vi "A Star Plan.vi"(8 "error in (no error)":errorcluster, 9 "goal reference":refnum<data-value>, 10 "start reference":refnum<data-value>, 11 "map reference in":refnum<data-value>) -> (0 "error out":errorcluster, 1 "no valid path exists":bool, 2 "path references":refnum<data-value>[](array[refnum]), 4 "path cost":dbl)   [LabVIEW 2017, in "NI_Robotics_Navigation .lvlib"]
doc: "Plans a least-cost path through a static map to a <B>goal reference</B> within a map. Use this VI to return a single, optimal path."
uses:
  <vilib>/robotics/Navigation/NI_Robotics_Navigation .lvlib
  <vilib>/robotics/Navigation/shared/MapNode/AbstractAstarNode/NI_Robotics_AbstractAstarNode.lvclass
  c:/Program Files (x86)/National Instruments/LabVIEW 2017/vi.lib/robotics/Navigation/shared/MapNode/AbstractMapNode/NI_Robotics_AbstractMapNode.lvclass
  <vilib>/robotics/Navigation/shared/WorldMap/AbstractWorldMap/NI_Robotics_AbstractWorldMap.lvclass
  <vilib>/robotics/Navigation/shared/Priority Queue/Open List Element.ctl
  <vilib>/robotics/Navigation/shared/MapNode/AbstractMapNode/NI_Robotics_AbstractMapNode.lvclass
  <vilib>/robotics/Navigation/Astar/Visited List Element.ctl
  <vilib>/robotics/Navigation/shared/Priority Queue/NI_Robotics_Priority Queue.lvclass
panel:
  out "num states":i32
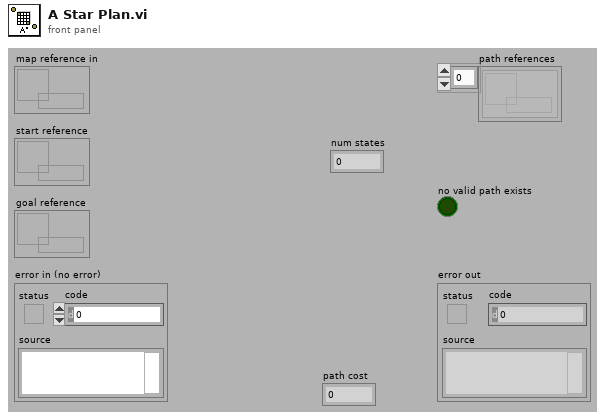
[diagram p1: front panel]
types:
  T1 = typedef "NI_Robotics_Priority Queue.lvclass/Open List Element.ctl" = cluster{"f":dbl, "g":dbl, "node Ref":refnum<data-value>}
  T2 = typedef "NI_Robotics_Navigation .lvlib/Visited List Element.ctl" = cluster{"Best cost to state":dbl, "Back pointer":refnum<data-value>}
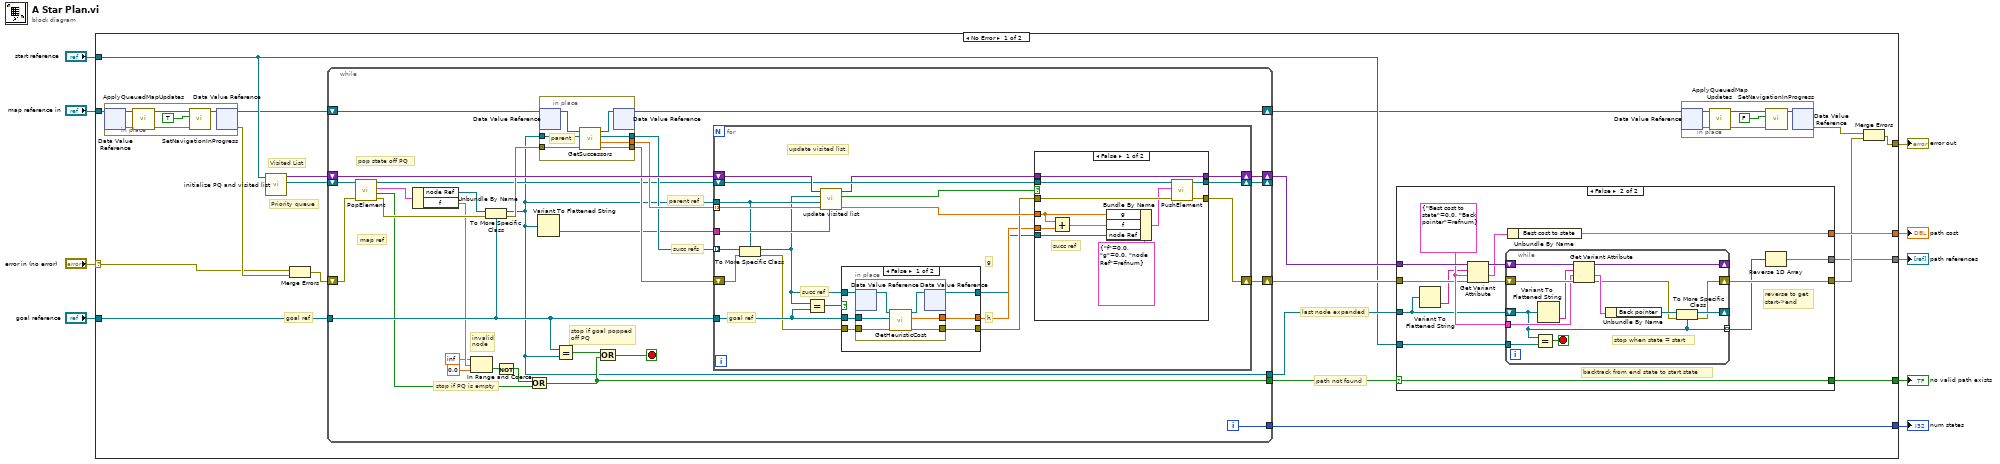
[diagram p0: block diagram]
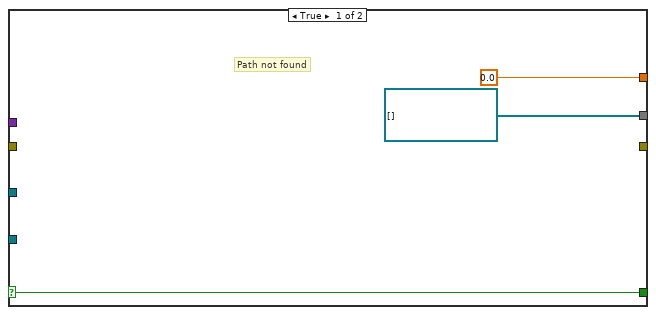
[diagram p2: hidden frame]
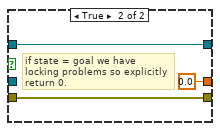
[diagram p3: hidden frame]
diagram:
  n1 = case shown="No Error" "error in (no error)" {
    selector: "error in (no error)" -> [w10 w158]
    tunnel: [w28 _] -> w9
    tunnel: "goal reference" -> [w23 _]
    tunnel: "start reference" -> [w22 _]
    tunnel: "map reference in" -> [w21 _]
    tunnel: [w15 w158] -> w5
    tunnel: [w13 _] -> w4
    tunnel: [w12 _] -> w3
    tunnel: [w11 _] -> w2
    frame No Error {
      # "goal ref"
      # "last node expanded"
      # "path not found"
      # "Priority queue"
      # "Visited List"
      n2 = in-place {
        n3 = in-place-dvr #1(w21) -> (w42:refnum<class "NI_Robotics_AbstractWorldMap.lvclass">, w41:errorcluster)
        n4 = call-dynamic "ApplyQueuedMapUpdates.vi"("error in (no error)"=w41, "AbstractWorldMap in"=w42) -> ("error out"=w38:errorcluster, "AbstractWorldMap out"=w40:refnum<class "NI_Robotics_AbstractWorldMap.lvclass">)  [unwired: 8 in]
        n5 = call-dynamic "SetNavigationInProgress.vi"("error in (no error)"=w38, "navigation in progress"=TRUE ("Navigation in Progress"), "AbstractWorldMap in"=w40) -> ("AbstractWorldMap out"=w39:refnum<class "NI_Robotics_AbstractWorldMap.lvclass">)  [unwired: 7 in, 1 out]
        n6 = in-place-dvr #1(w39) -> (w20:refnum<data-value>, w17:errorcluster)
      }
      n7 = call <vilib>:"initialize PQ and visited list.vi"("start state"=w22) -> ("Astar Open List out"=w24:refnum<class "NI_Robotics_Priority Queue.lvclass">, "visited list"=w30:variant)  [unwired: 9 out]
      n8 = Merge Errors(w10, w17) -> (w18:errorcluster)
      n9 = while {
        shift-right: [w97] -> _
        shift-left: w24 -> [w95]
        shift-right: [w99] -> w27
        shift-left: w30 -> [w101]
        tunnel: [w74] -> w26
        tunnel: w23 -> [w83]
        shift-right: [w98] -> w29
        shift-left: w18 -> [w94]
        tunnel: [w80] -> w25
        shift-right: [w82] -> w19
        shift-left: w20 -> [w84]
        tunnel: [w73] -> w12
        i -> [w73]
        stop <- w96 stop-if-true
        # "parent ref"
        # "invalid\nnode"
        # "map ref"
        # "succ refs"
        # "stop if goal popped\noff PQ"
        # "stop if PQ is empty"
        # "pop state off PQ"
        n10 = call <vilib>:"PopElement.vi"("error in (no error)"=w94, "Astar Open List in"=w95) -> ("error out"=w92:errorcluster, "empty"=w81:bool, "open list element"=w93:T1, "Astar Open List out"=w87:refnum<class "NI_Robotics_Priority Queue.lvclass">)  [unwired: 6 in]
        n11 = Unbundle By Name(w93) -> ("node Ref"=w85:refnum<data-value>, "f"=w79:dbl)
        n12 = In Range and Coerce(upper limit=inf, x=w79, lower limit=0.0) -> (In Range?=w75:bool)  [unwired: 1 out]
        n13 = To More Specific Class(target class=w83, reference=w85, error in=w92) -> (specific class reference=w74:refnum<data-value>, error out=w91:errorcluster)
        n14 = Not(x=w75) -> (.not. x?=w76:bool)
        n15 = Or(x=w76, y=w81) -> (x .or. y?=w80:bool)
        n16 = Variant To Flattened String(Variant=w74) -> (data string=w86:string)  [unwired: 1 out]
        n17 = in-place {
          in-place-border: w91 -> [w108]
          in-place-border: [w107] -> w90
          in-place-border: [w106] -> w89
          in-place-border: [w105] -> w88
          in-place-border: w74 -> [w102]
          # "parent"
          n18 = in-place-dvr #2(w84) -> (w104:refnum<class "NI_Robotics_AbstractWorldMap.lvclass">)  [unwired: 1 out]
          n19 = call-dynamic "GetSuccessors.vi"("error in (no error)"=w108, "AbstractMapNode Ref"=w102, "WorldMap in"=w104) -> ("error out"=w107:errorcluster, "EdgeCost"=w106:dbl[], "Successors"=w105:refnum<data-value>[], "WorldMap out"=w103:refnum<class "NI_Robotics_AbstractWorldMap.lvclass">)  [unwired: 5 in]
          n20 = in-place-dvr #2(w103) -> (w82:refnum<data-value>)  [unwired: 1 out]
        }
        n21 = Equal?(x=w83, y=w74) -> (x = y?=w100:bool)
        n22 = Or(x=w100, y=w80) -> (x .or. y?=w96:bool)
        n23 = for {
          shift-right: [w124] -> w97
          shift-left: w87 -> [w125]
          shift-right: [w109] -> w99
          shift-left: w101 -> [w128]
          tunnel: w88 -> [w122] mode=indexing
          tunnel: w89 -> [w118] mode=indexing
          tunnel: w86 -> [w119]
          tunnel: w83 -> [w113]
          shift-right: [w123] -> w98
          shift-left: w90 -> [w112]
          tunnel: w74 -> [w117]
          # "succ ref"
          # "goal ref"
          # "h"
          # "g"
          # "update visited list"
          n24 = To More Specific Class(target class=w117, reference=w122, error in=w112) -> (specific class reference=w114:refnum<data-value>, error out=w111:errorcluster)
          n25 = Equal?(x=w114, y=w113) -> (x = y?=w115:bool)
          n26 = call <vilib>:"update visited list.vi"("previous node string"=w119, "edge cost"=w118, "previous node"=w117, "current node"=w114, "visited list in"=w128) -> ("path cost"=w126:dbl, "discarded"=w127:bool, "visited list out"=w110:variant)  [unwired: 4 out]
          n27 = case shown="False" w115 {
            tunnel: w113 -> [w134 _]
            tunnel: w111 -> [w133 w142]
            tunnel: [w132 w142] -> w121
            tunnel: [w131 0.0 ("Hueristic Cost")] -> w120
            tunnel: w114 -> [w130 w143]
            tunnel: [w129 w143] -> w116
            frame False {
              n28 = in-place {
                in-place-border: w134 -> [w140]
                in-place-border: w133 -> [w139]
                in-place-border: [w138] -> w132
                in-place-border: [w137] -> w131
                n29 = in-place-dvr #3(w130) -> (w136:refnum<class "NI_Robotics_AbstractAstarNode.lvclass">)  [unwired: 1 out]
                n30 = call-dynamic "GetHeuristicCost.vi"("error in (no error)"=w139, "Goal NodeReference"=w140, "AbstractAstarNode in"=w136) -> ("error out"=w138:errorcluster, "hueristic cost"=w137:dbl, "AbstractAstarNode out"=w135:refnum<class "NI_Robotics_AbstractAstarNode.lvclass">)  [unwired: 6 in]
                n31 = in-place-dvr #3(w135) -> (w129:refnum<data-value>)  [unwired: 1 out]
              }
            }
            frame True {
              # "if state = goal we have locking problems so explicitly return 0."
            }
          }
          n32 = case shown="False" w127 {
            tunnel: w126 -> [w147 _]
            tunnel: w125 -> [w152 w156]
            tunnel: [w149 w156] -> w124
            tunnel: w120 -> [w148 _]
            tunnel: w116 -> [w153 _]
            tunnel: w121 -> [w151 w157]
            tunnel: [w150 w157] -> w123
            tunnel: w110 -> [w146 w155]
            tunnel: [w146 w155] -> w109
            frame False {
              # "succ ref"
              n33 = Add(x=w147, y=w148) -> (x+y=w154:dbl)
              n34 = Bundle By Name(cluster=T1 {"f"=0.0, "g"=0.0, "node Ref"=refnum} ("Open List Element"), "g"=w147, "f"=w154, "node Ref"=w153) -> (w145:T1)
              n35 = call <vilib>:"PushElement.vi"("error in (no error)"=w151, "open list element"=w145, "Astar Open List in"=w152) -> ("error out"=w150:errorcluster, "Astar Open List out"=w149:refnum<class "NI_Robotics_Priority Queue.lvclass">)  [unwired: 7 in]
            }
            frame True {
              # "There is a better path\nalready known"
            }
          }
        }
      }
      n36 = case shown="False" w25 {
        selector: w25 -> [w43 w46]
        tunnel: w22 -> [_ w59]
        tunnel: w29 -> [_ w51]
        tunnel: [refnum<data-value>[] [] w58] -> w11
        tunnel: [_ w57] -> w14
        tunnel: [0.0 ("Best cost to state") w52] -> w28
        tunnel: w27 -> [_ w56]
        tunnel: w26 -> [_ w47]
        tunnel: [w43 w46] -> w13
        frame True {
          # "Path not found"
        }
        frame False {
          w54 = T2 {"Best cost to state"=0.0, "Back pointer"=refnum} ("Visited Element")
          # "backtrack from end state to start state"
          # "reverse to get\nstart->end"
          n37 = Variant To Flattened String(Variant=w47) -> (data string=w49:string)  [unwired: 1 out]
          n38 = Get Variant Attribute(Variant=w56, name=w49, default value (empty Variant)=w54, error in=w51) -> (duplicate Variant=w55:variant, value=w53:T2, error out=w50:errorcluster)  [unwired: 1 out]
          n39 = while {
            shift-right: [w64] -> _
            shift-left: w47 -> [w62]
            tunnel: w59 -> [w63]
            shift-right: [w68] -> _
            shift-left: w55 -> [w71]
            shift-right: [w61] -> w57
            shift-left: w50 -> [w70]
            tunnel: w54 -> [w67]
            tunnel: [w62] -> w48 mode=indexing
            stop <- w72 stop-if-true
            # "stop when state = start"
            n40 = Equal?(x=w62, y=w63) -> (x = y?=w72:bool)
            n41 = Variant To Flattened String(Variant=w62) -> (data string=w66:string)  [unwired: 1 out]
            n42 = Get Variant Attribute(Variant=w71, name=w66, default value (empty Variant)=w67, error in=w70) -> (duplicate Variant=w68:variant, value=w69:T2, error out=w60:errorcluster)  [unwired: 1 out]
            n43 = Unbundle By Name(w69) -> ("Back pointer"=w65:refnum<data-value>)
            n44 = To More Specific Class(target class=w62, reference=w65, error in=w60) -> (specific class reference=w64:refnum<data-value>, error out=w61:errorcluster)
          }
          n45 = Unbundle By Name(w53) -> ("Best cost to state"=w52:dbl)
          n46 = Reverse 1D Array(array=w48) -> (reversed array=w58:refnum<data-value>[])
        }
      }
      n47 = in-place {
        n48 = in-place-dvr #4(w19) -> (w36:refnum<class "NI_Robotics_AbstractWorldMap.lvclass">, w35:errorcluster)
        n49 = call-dynamic "ApplyQueuedMapUpdates.vi"("error in (no error)"=w35, "AbstractWorldMap in"=w36) -> ("error out"=w32:errorcluster, "AbstractWorldMap out"=w34:refnum<class "NI_Robotics_AbstractWorldMap.lvclass">)  [unwired: 8 in]
        n50 = call-dynamic "SetNavigationInProgress.vi"("error in (no error)"=w32, "navigation in progress"=FALSE ("Navigation in Progress"), "AbstractWorldMap in"=w34) -> ("AbstractWorldMap out"=w33:refnum<class "NI_Robotics_AbstractWorldMap.lvclass">)  [unwired: 7 in, 1 out]
        n51 = in-place-dvr #4(w33) -> (w16:errorcluster)  [unwired: 1 out]
      }
      n52 = Merge Errors(w16, w14) -> (w15:errorcluster)
    }
    frame Error {
    }
  }
  "error out" <- w5
  "path cost" <- w9
  "path references" <- w2
  "no valid path exists" <- w4
  "num states" <- w3
